vi "Speed_Computation.vi"(10 "Speed":u8 format="%x", 11 "identifier":u8 format="%x") -> (2 "output cluster":T1 {"payload" format="%x"; "timestamp" format="%<%I:%M:%S%8u %p\n%x>T"; "identifier" format="%x"})   [LabVIEW 2015]
uses:
  <vilib>/Stratom, Inc/X-CAN for myRIO (API)/X-CAN Class/Type Definitions/CANFrame.ctl
  <vilib>/Stratom, Inc/X-CAN for myRIO (API)/X-CAN Class/X-CAN.lvclass
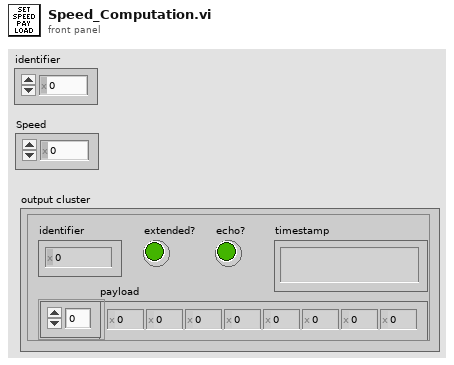
[diagram p1: front panel]
types:
  T1 = typedef "X-CAN.lvclass/CANFrame.ctl" = cluster{"identifier":u32, "extended?":bool, "echo?":bool, "payload":u8[], "timestamp":timestamp}
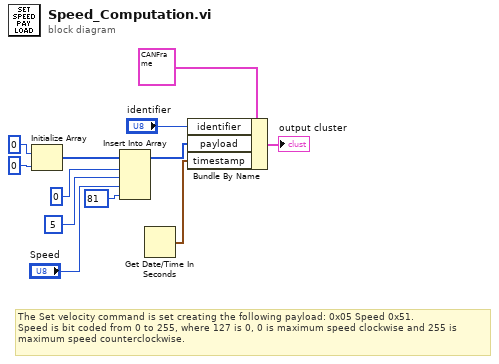
[diagram p0: block diagram]
diagram:
  # "The Set velocity command is set creating the following payload: 0x05 Speed 0x51.\nSpeed is bit coded from 0 to 255, where 127 is 0, 0 is maximum speed clockwise and 255 is\nmaximum speed counterclockwise."
  n1 = Initialize Array(u16 0 ("element"), 0 ("dimension size")) -> (w8:u16[])
  n2 = Insert Into Array(array=w8, index=0, new element #1=u8 5 ("new element/subarray"), new element #2="Speed", new element #3=u8 81 ("new element/subarray")) -> (w5:u16[])
  n3 = Get Date/Time In Seconds() -> (seconds since 1Jan1904=w12:timestamp)
  n4 = Bundle By Name(cluster=T1 {"identifier"=0, "extended?"=FALSE, "echo?"=FALSE, "payload"=[], "timestamp"=timestamp(0 s since 1904-01-01)} ("CAN Frame"), "identifier"="identifier", "payload"=w5, "timestamp"=w12) -> (→"output cluster":T1)
